vi "Main.vi"() -> ()   [LabVIEW 2014]
doc: "Use this template to build a simple state machine design pattern. Each state executes code and determines which state to transition to."
uses:
  controls/State.ctl
  controls/Data.ctl
panel:
  in  "Gerar nova onda":bool
  in  "Salvar onda":bool
  in  "Histórico de ondas":bool
  in  "Adquirir dados":bool
  in  "Sair":bool
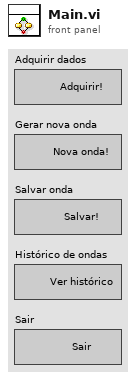
[diagram p1: front panel]
types:
  T1 = typedef "Data.ctl" = cluster{"Boolean <Replace Me>":bool, "String <Replace Me>":string, "Numeric <Replace Me>":dbl}
  T2 = typedef "State.ctl" = enum16{"Inicializar", "Aguardar evento", "Adquirir dados", "Gerar nova onda", "Salvar onda", "Histórico de ondas", "Sair"}
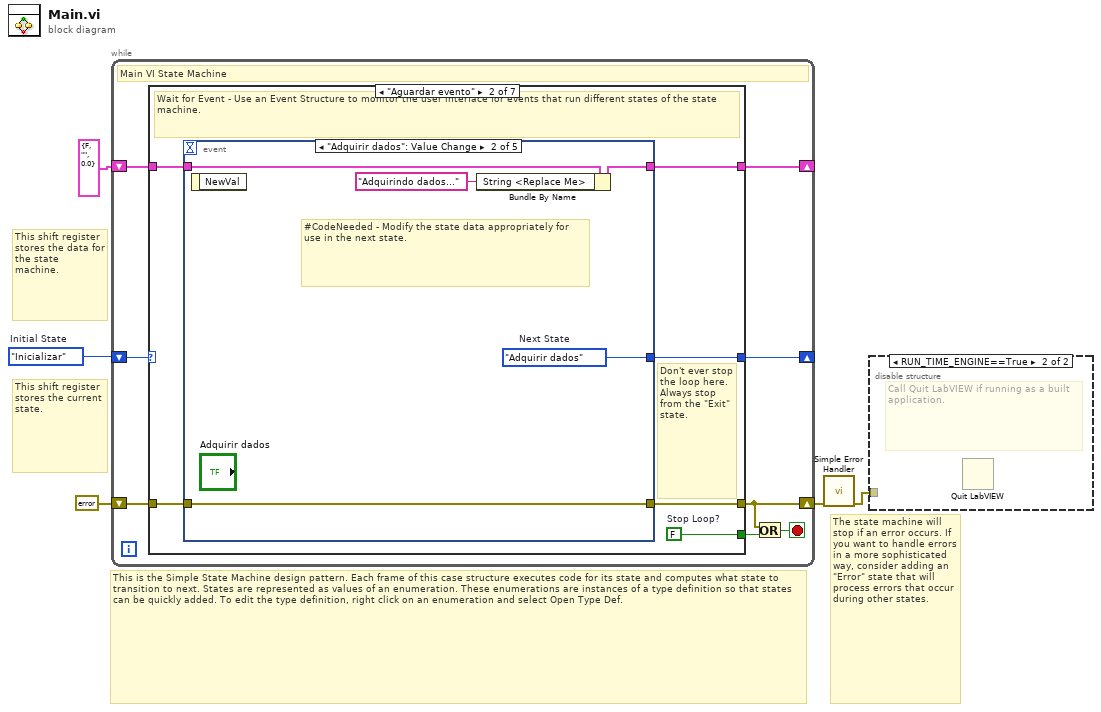
[diagram p0: block diagram]
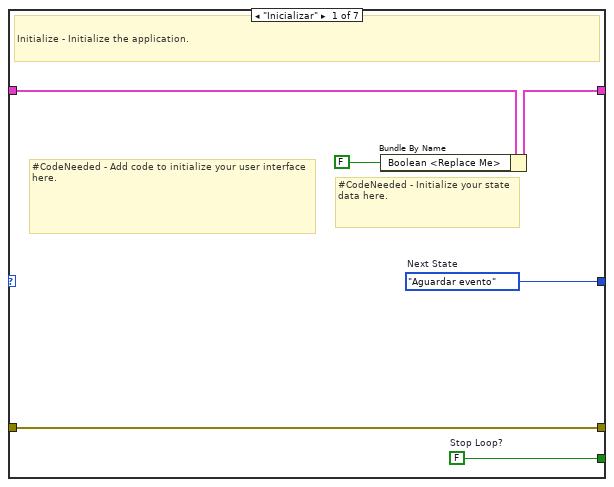
[diagram p3: hidden frame]
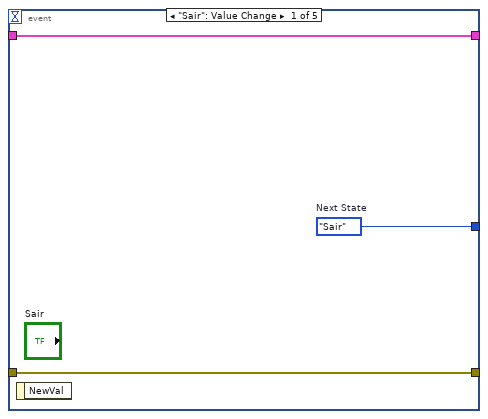
[diagram p4: hidden frame]
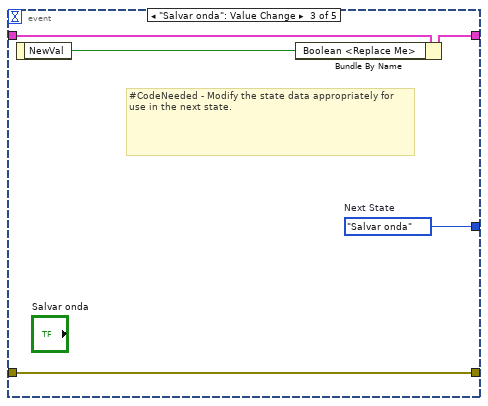
[diagram p5: hidden frame]
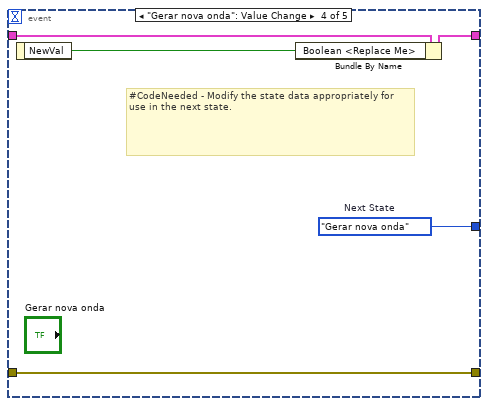
[diagram p6: hidden frame]
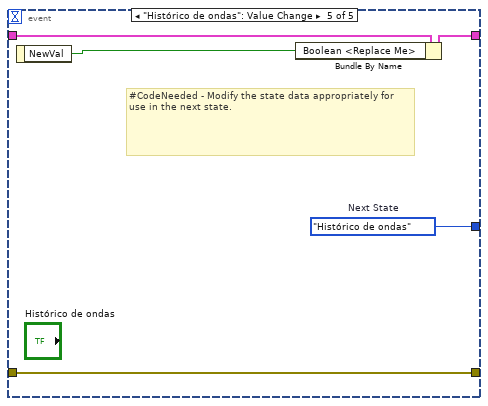
[diagram p7: hidden frame]
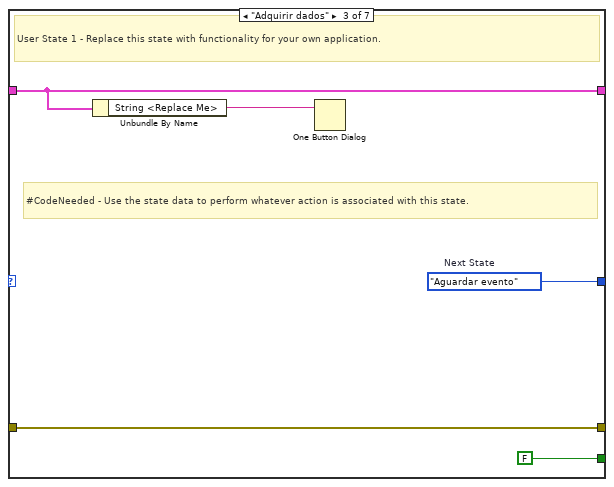
[diagram p8: hidden frame]
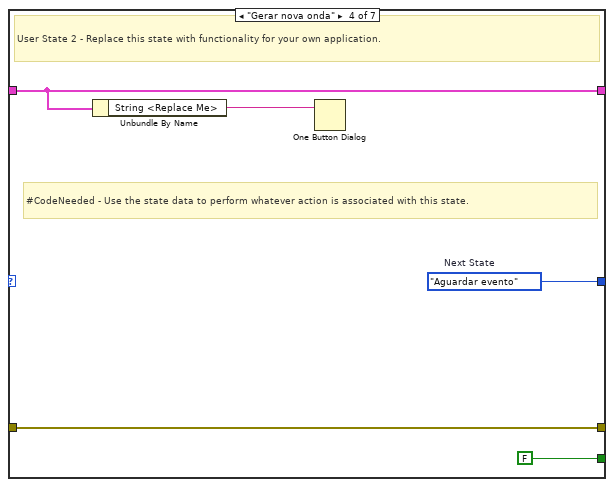
[diagram p9: hidden frame]
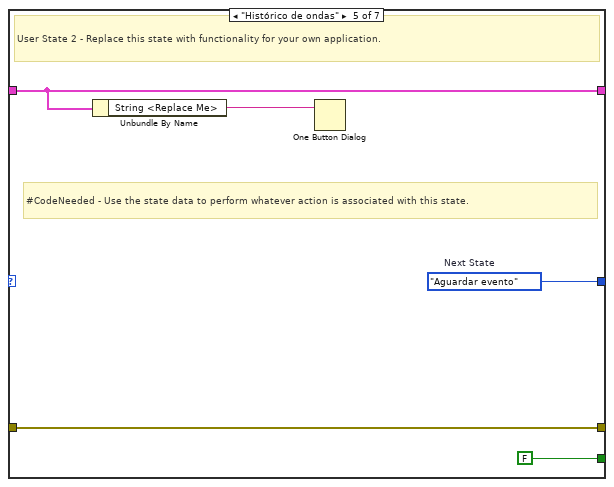
[diagram p10: hidden frame]
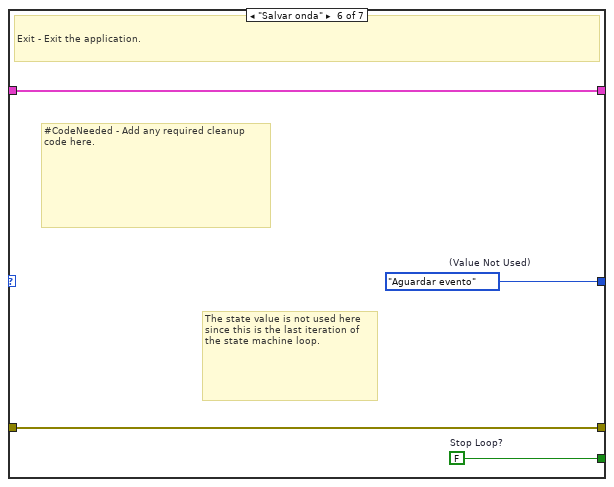
[diagram p11: hidden frame]
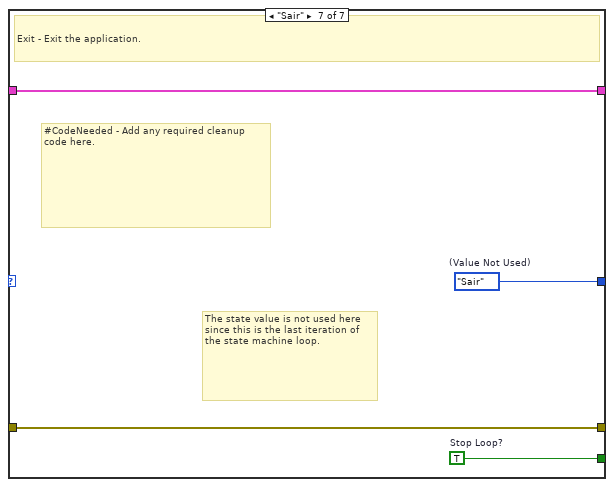
[diagram p12: hidden frame]
diagram:
  w5 = State."Inicializar"  # Initial State
  # "The state machine will stop if an error occurs. If you want to handle errors in a more sophisticated way, consider adding an \"Error\" state that will process errors that occur during other states."
  # "This shift register stores the data for the state machine."
  # "This is the Simple State Machine design pattern. Each frame of this case structure executes code for its state and computes what state to transition to next. States are represented as values of an enumeration. These enumerations are instances of a type definition so that states can be quickly added. To edit the type definition, right click on an enumeration and select Open Type Def."
  # "This shift register stores the current state."
  n1 = while {
    shift-right: [w12] -> _
    shift-left: w5 -> [w13]
    shift-right: [w10] -> _
    shift-left: T1 {"Boolean <Replace Me>"=FALSE, "String <Replace Me>"="", "Numeric <Replace Me>"=0.0} ("Data") -> [w11]
    shift-right: [w6] -> w2
    shift-left: errorcluster {"status"=FALSE, "code"=0, "source"=""} ("error constant") -> [w9]
    stop <- w7 stop-if-true
    # "Main VI State Machine"
    n2 = case shown="\"Aguardar evento\"" w13 {
      tunnel: [w19 w25 w53 w58 w63 w67 w71] -> w12
      tunnel: [w18 w24 FALSE ("Stop Loop?") FALSE ("Stop Loop?") FALSE ("Stop Loop?") w65 w69] -> w8
      tunnel: w11 -> [w17 w23 w51 w56 w61 w66 w70]
      tunnel: [w16 w22 w51 w56 w61 w66 w70] -> w10
      tunnel: w9 -> [w14 w21 w49 w54 w59 w64 w68]
      tunnel: [w14 w20 w49 w54 w59 w64 w68] -> w6
      frame "Inicializar" {
        w18 = FALSE  # Stop Loop?
        w19 = State."Aguardar evento"  # Next State
        # "#CodeNeeded - Initialize your state data here."
        # "#CodeNeeded - Add code to initialize your user interface here."
        # "Initialize - Initialize the application."
        n3 = Bundle By Name(cluster=w17, "Boolean <Replace Me>"=FALSE ("Replace_Me_Boolean")) -> (w16:T1)
      }
      frame "Aguardar evento" {
        w24 = FALSE  # Stop Loop?
        # "Don't ever stop the loop here. Always stop from the \"Exit\" state."
        # "Wait for Event - Use an Event Structure to monitor the user interface for events that run different states of the state machine."
        n4 = event shown="[1] \"Adquirir dados\": Value Change" {
          selector: _ -> [_ _ _ _ _]
          dyn-events: _ -> [_ _ _ _ _]
          timeout: _ -> [_ _ _ _ _]
          tunnel: [w28 w33 w38 w43 w48] -> w25
          tunnel: w23 -> [w27 w32 w37 w42 w47]
          tunnel: [w27 w31 w36 w41 w46] -> w22
          tunnel: w21 -> [w26 w30 w35 w40 w45]
          tunnel: [w26 w30 w35 w40 w45] -> w20
          event "Sair": Value Change {
            w28 = State."Sair"  # Next State
            n5 = event-data() -> ()  [unwired: 1 in, 1 out]
          }
          event "Adquirir dados": Value Change {
            w33 = State."Adquirir dados"  # Next State
            # "#CodeNeeded - Modify the state data appropriately for use in the next state."
            n6 = event-data() -> ()  [unwired: 1 in, 1 out]
            n7 = Bundle By Name(cluster=w32, "String <Replace Me>"="Adquirindo dados...") -> (w31:T1)
          }
          event "Salvar onda": Value Change {
            w38 = State."Salvar onda"  # Next State
            # "#CodeNeeded - Modify the state data appropriately for use in the next state."
            n8 = event-data() -> ("NewVal"=w34:bool)  [unwired: 1 in]
            n9 = Bundle By Name(cluster=w37, "Boolean <Replace Me>"=w34) -> (w36:T1)
          }
          event "Gerar nova onda": Value Change {
            w43 = State."Gerar nova onda"  # Next State
            # "#CodeNeeded - Modify the state data appropriately for use in the next state."
            n10 = event-data() -> ("NewVal"=w39:bool)  [unwired: 1 in]
            n11 = Bundle By Name(cluster=w42, "Boolean <Replace Me>"=w39) -> (w41:T1)
          }
          event "Histórico de ondas": Value Change {
            w48 = State."Histórico de ondas"  # Next State
            # "#CodeNeeded - Modify the state data appropriately for use in the next state."
            n12 = event-data() -> ("NewVal"=w44:bool)  [unwired: 1 in]
            n13 = Bundle By Name(cluster=w47, "Boolean <Replace Me>"=w44) -> (w46:T1)
          }
        }
      }
      frame "Adquirir dados" {
        w53 = State."Aguardar evento"  # Next State
        # "#CodeNeeded - Use the state data to perform whatever action is associated with this state."
        # "User State 1 - Replace this state with functionality for your own application."
        n14 = Unbundle By Name(w51) -> ("String <Replace Me>"=w50:string)
        n15 = One Button Dialog(message=w50) -> ()  [unwired: 1 in, 1 out]
      }
      frame "Gerar nova onda" {
        w58 = State."Aguardar evento"  # Next State
        # "#CodeNeeded - Use the state data to perform whatever action is associated with this state."
        # "User State 2 - Replace this state with functionality for your own application."
        n16 = Unbundle By Name(w56) -> ("String <Replace Me>"=w55:string)
        n17 = One Button Dialog(message=w55) -> ()  [unwired: 1 in, 1 out]
      }
      frame "Histórico de ondas" {
        w63 = State."Aguardar evento"  # Next State
        # "#CodeNeeded - Use the state data to perform whatever action is associated with this state."
        # "User State 2 - Replace this state with functionality for your own application."
        n18 = Unbundle By Name(w61) -> ("String <Replace Me>"=w60:string)
        n19 = One Button Dialog(message=w60) -> ()  [unwired: 1 in, 1 out]
      }
      frame "Salvar onda" {
        w65 = FALSE  # Stop Loop?
        w67 = State."Aguardar evento"  # (Value Not Used)
        # "#CodeNeeded - Add any required cleanup code here."
        # "The state value is not used here since this is the last iteration of the state machine loop."
        # "Exit - Exit the application."
      }
      frame "Sair" {
        w69 = TRUE  # Stop Loop?
        w71 = State."Sair"  # (Value Not Used)
        # "#CodeNeeded - Add any required cleanup code here."
        # "The state value is not used here since this is the last iteration of the state machine loop."
        # "Exit - Exit the application."
      }
    }
    n20 = Or(x=w6, y=w8) -> (x .or. y?=w7:bool)
  }
  n21 = call <vilib>:"Simple Error Handler.vi"("error in (no error)"=w2) -> ("error out"=w1:errorcluster)  [unwired: 4 in, 4 out]
  n22 = disable-structure shown="RUN_TIME_ENGINE==True" {
    disable-tunnel: w1 -> [_ _]
    frame condition #0 (active) {
    }
    frame condition #1 {
      # "Call Quit LabVIEW if running as a built application."
      n23 = Quit LabVIEW() -> ()  [unwired: 1 in]
    }
  }
